vi "Create Channel Name Cluster.vi"(8 "error in":errorcluster, 9 "Numeric":u8, 10 "Cluster":variant, 11 "Instance Name":string) -> (0 "error out":errorcluster, 3 "Data Channel Name":string)   [LabVIEW 2023, in "Utilities.lvlib"]
uses:
  Utilities.lvlib
  <vilib>/Utility/Data Type/NI_Data Type.lvlib
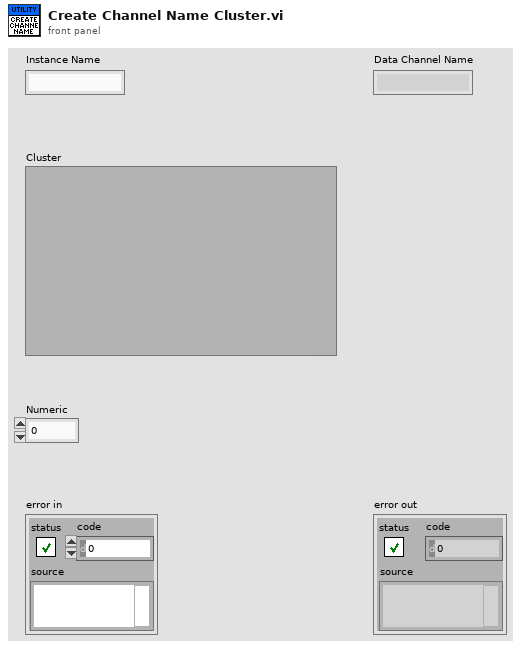
[diagram p1: front panel]
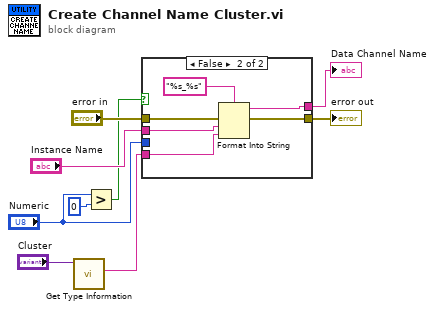
[diagram p0: block diagram]
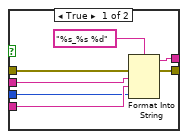
[diagram p2: hidden frame]
diagram:
  n1 = call <vilib>:"Get Type Information.vi"("variant"="Cluster") -> ("name"=w5:string)  [unwired: 6 in, 4 out]
  n2 = Greater?(x="Numeric", y=u8 0 ("x")) -> (0:w1:bool)
  n3 = case shown="False" w1 {
    tunnel: "error in" -> [w15 w21]
    tunnel: "Instance Name" -> [w14 w20]
    tunnel: w5 -> [w13 w19]
    tunnel: "Numeric" -> [w12 _]
    tunnel: [w11 w18] -> w3
    tunnel: [w10 w17] -> w2
    frame True {
      n4 = Format Into String(format string="%s_%s %d", error in=w15, w14, w13, w12) -> (resulting string=w11:string, error out=w10:errorcluster)  [unwired: 1 in]
    }
    frame False {
      n5 = Format Into String(format string="%s_%s", error in=w21, w20, w19) -> (resulting string=w18:string, error out=w17:errorcluster)  [unwired: 1 in]
    }
  }
  "error out" <- w2
  "Data Channel Name" <- w3
